vi "read_sense.vi"(1 "VISA session (for class)":refnum<visa-resource-name>) -> (0 "sense":string)   [LabVIEW 2015]
doc: "This VI reads the sensetivity parameter of the Lock-In."
panel:
  out "SEN":i32
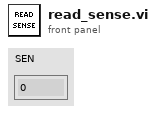
[diagram p1: front panel]
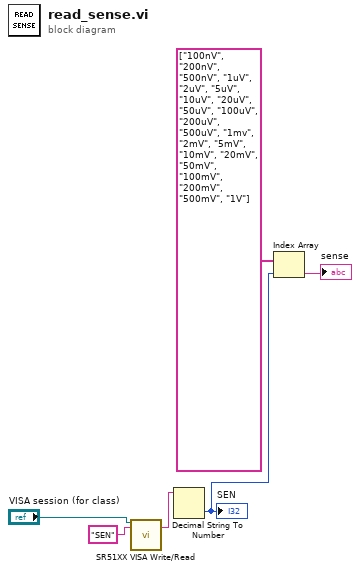
[diagram p0: block diagram]
diagram:
  n1 = call "SR51XX VISA Write/Read"("VISA session (for class)"="VISA session (for class)", "Write Command String"="SEN") -> ("Response 1"=w6:string)  [unwired: 6 in, 11 out]
  n2 = Decimal String To Number(string=w6) -> (number=w3:i32)  [unwired: 2 in, 1 out]
  "SEN" <- w3
  n3 = Index Array(array=string[] ["100nV", "200nV", "500nV", "1uV", "2uV", "5uV", "10uV", "20uV", "50uV", "100uV", "200uV", "500uV", "1mv", "2mV", "5mV", "10mV", "20mV", "50mV", "100mV", "200mV", "500mV", "1V"], index=w3) -> (element=→"sense":string)
